vi "First Order Lag Filter (1D DBL).vi"(1 "k (1)":dbl=1.0, 2 "Raw Values in":dbl[](array[numeric]), 4 "Prev Filtered Vals (Optional)":dbl[](array[numeric])) -> (6 "Filtered Values out":dbl[](array[numeric]))   [LabVIEW 2018, in "RT - Analysis.lvlib"]
doc: "Performs a 1st Order Lag on a single value following the equation:\n<B>NewFilteredVal = k * RawVal + (1 - k) * OldFilteredVal</B>"
uses:
  RT - Analysis.lvlib
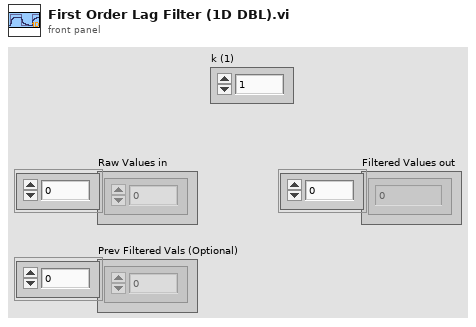
[diagram p1: front panel]
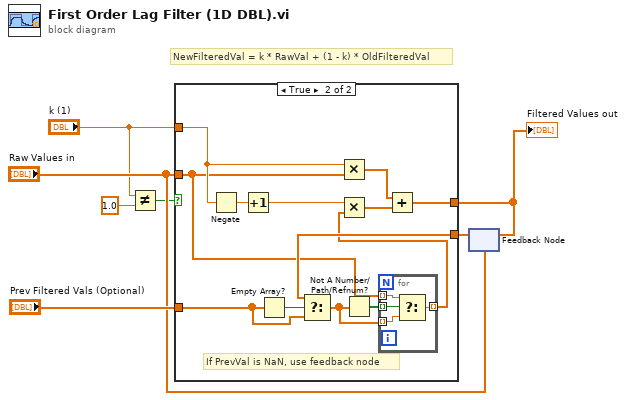
[diagram p0: block diagram]
diagram:
  # "NewFilteredVal = k * RawVal + (1 - k) * OldFilteredVal"
  n1 = Not Equal?(x="k (1)", y=1.0) -> (x != y?=w3:bool)
  n2 = feedback #1("Raw Values in") -> (w6:dbl[])
  n3 = case shown="True" w3 {
    tunnel: [w8 w21] -> w7
    tunnel: "k (1)" -> [_ w18]
    tunnel: "Raw Values in" -> [w8 w11]
    tunnel: w6 -> [_ w14]
    tunnel: "Prev Filtered Vals (Optional)" -> [_ w13]
    frame False {
    }
    frame True {
      # "If PrevVal is NaN, use feedback node"
      n4 = Negate(x=w18) -> (-x=w19:dbl)
      n5 = Increment(x=w19) -> (x+1=w20:dbl)
      n6 = Empty Array?(array=w13) -> (empty?=w15:bool)
      n7 = Select(t=w14, s=w15, f=w13) -> (s? t:f=w10:dbl[])
      n8 = Multiply(x=w18, y=w11) -> (x*y=w16:dbl[])
      n9 = Not A Number/Path/Refnum?(number/path/refnum=w10) -> (NaN/Path/Refnum?=w12:bool[])
      n10 = for {
        tunnel: w12 -> [w25] mode=indexing
        tunnel: w10 -> [w24] mode=indexing
        tunnel: w11 -> [w23] mode=indexing
        tunnel: [w22] -> w9 mode=indexing
        n11 = Select(t=w23, s=w25, f=w24) -> (s? t:f=w22:dbl)
      }
      n12 = Multiply(x=w20, y=w9) -> (x*y=w17:dbl[])
      n13 = Add(x=w16, y=w17) -> (x+y=w21:dbl[])
    }
  }
  "Filtered Values out" <- w7
  n14 = feedback-in #1(w7) -> ()
